vi "Config_Pulses_Tomography_v1.vi"(7 "init file iterator":u8, 8 "error in":errorcluster, 10 "Config files paths":T1={"ZI config file (.ini)"="Tomography_v1_config_dir\\Zurich_params.ini", "Keithley config file (.ini)"="Tomography_v1_config_dir\\Keithley_params.ini", "Arduino config file (.ini)"="Tomography_v1_config_dir\\pulse_sequence_dir\\"}, 11 "Resources in":T2 {"ZI ModHandle"."ModHandle" format="0x%08x"; "ZI ModHandle"."Conn" format="0x%08x"; "ZI Handle"."Handle" format="0x%08x"; "ZI Handle"."Conn" format="0x%08x"}) -> (0 "error out":errorcluster, 1 "Pulse sequence":T5[](array[typedef]) {"channel" min=2 max=13 step=1}, 2 "Init States":T8, 3 "Resources out":T2 {"ZI ModHandle"."ModHandle" format="0x%08x"; "ZI ModHandle"."Conn" format="0x%08x"; "ZI Handle"."Handle" format="0x%08x"; "ZI Handle"."Conn" format="0x%08x"}, 5 "Config files paths (single)":T1={"ZI config file (.ini)"="Config_Ver_1\\Zurich_params.ini", "Keithley config file (.ini)"="Config_Ver_1\\Keithley_params.ini", "Arduino config file (.ini)"="Config_Ver_1\\pulse_sequence.ini"})   [LabVIEW 2021]
uses:
  Ver_1/Config_File_Paths.ctl
  Ver_1/Resources.ctl
  <instrlib>/Zurich Instruments LabOne/Public/ziTypeHandle.ctl
  <instrlib>/Zurich Instruments LabOne/Public/Modules/ziTypeModHandle.ctl
  Drivers/Arduino_Pulse_Generator/Configurate/Register_1.ctl
  Drivers/Arduino_Pulse_Generator/Configurate/Register_2.ctl
  Drivers/Arduino_Pulse_Generator/Configurate/Channel_Pulse_Stream.ctl
  <instrlib>/Zurich Instruments LabOne/Zurich Instruments LabOne.lvlib
panel:
  out "String":string
  out "x-y":u32
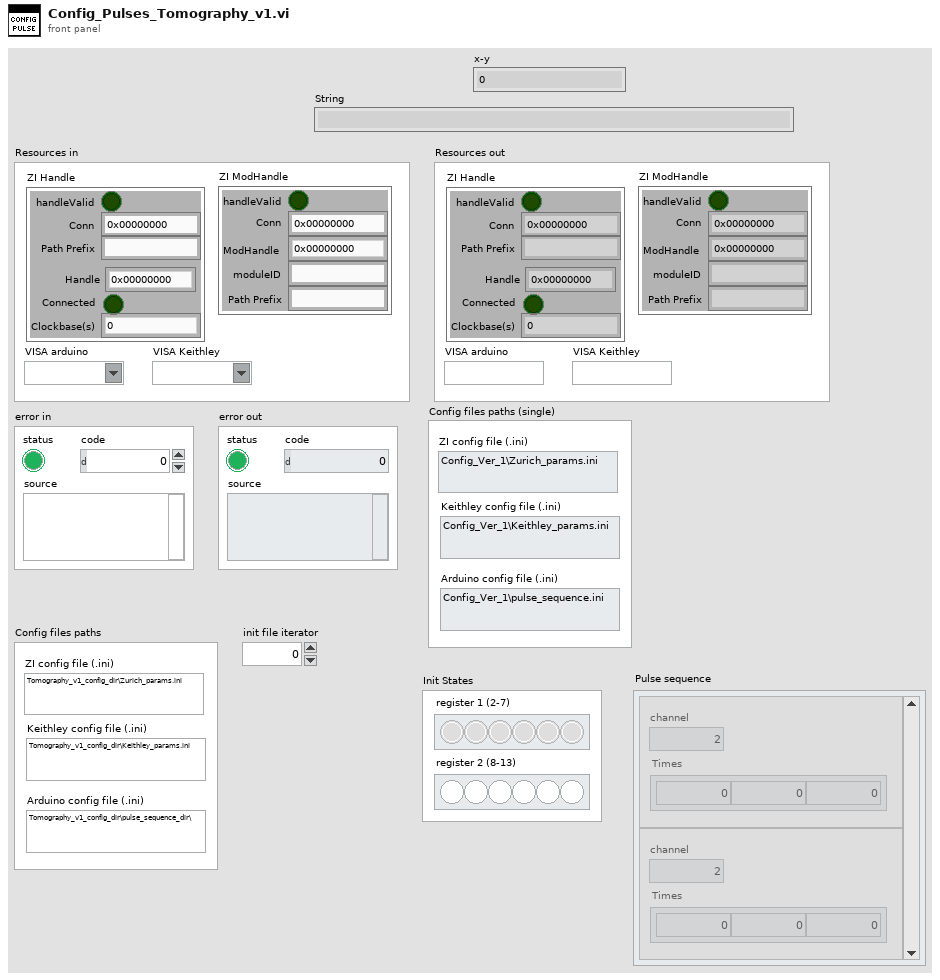
[diagram p1: front panel]
types:
  T1 = typedef "Config_File_Paths.ctl" = cluster{"ZI config file (.ini)":string, "Keithley config file (.ini)":string, "Arduino config file (.ini)":string}
  T2 = typedef "Resources.ctl" = cluster{"ZI Handle":T3, "ZI ModHandle":T4, "VISA arduino":refnum<visa-resource-name>, "VISA Keithley":refnum<visa-resource-name>}
  T3 = typedef "Zurich Instruments LabOne.lvlib/ziTypeHandle.ctl" = cluster{"handleValid":bool, "Conn":u64, "Path Prefix":string, "Handle":u64, "Connected":bool, "Clockbase(s)":dbl}
  T4 = typedef "Zurich Instruments LabOne.lvlib/ziTypeModHandle.ctl" = cluster{"handleValid":bool, "Conn":u64, "ModHandle":u64, "moduleID":string, "Path Prefix":string}
  T5 = typedef "Channel_Pulse_Stream.ctl" = cluster{"Times":dbl[], "channel":u8}
  T6 = typedef "Register_1.ctl" = bool[]
  T7 = typedef "Register_2.ctl" = bool[]
  T8 = cluster{"register 1 (2-7)":T6, "register 2 (8-13)":T7}
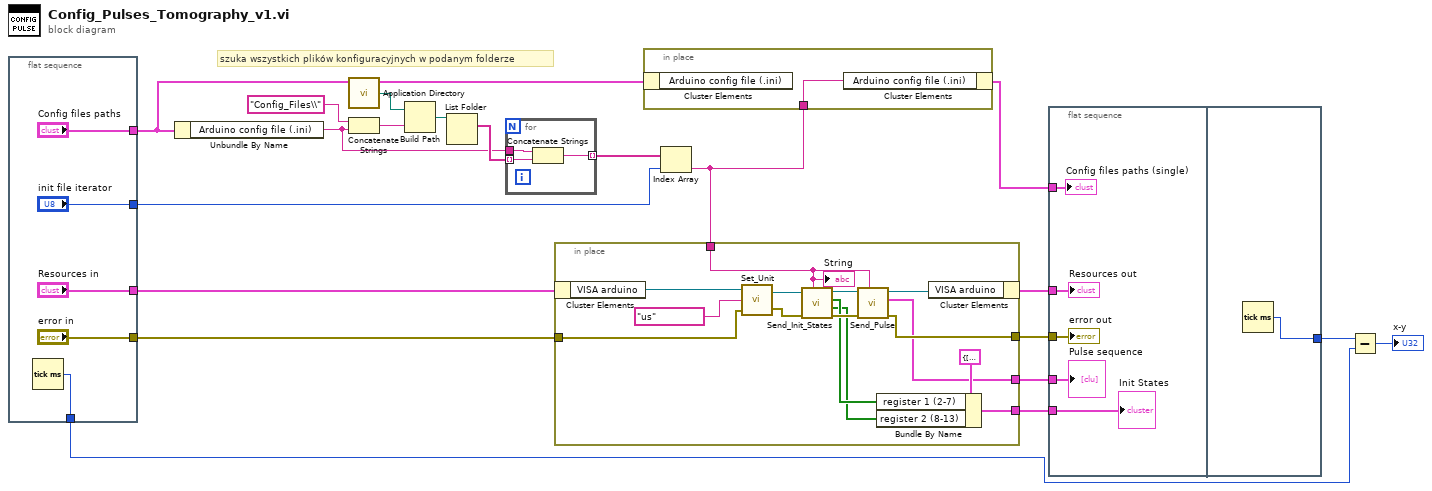
[diagram p0: block diagram]
diagram:
  # "szuka wszystkich plików konfiguracyjnych w podanym folderze"
  n1 = flat-sequence {
    tunnel: ["Config files paths"] -> w3
    tunnel: ["Resources in"] -> w14
    tunnel: ["init file iterator"] -> w12
    tunnel: ["error in"] -> w11
    tunnel: [w21] -> w5
    frame #0 {
      n2 = Tick Count (ms)() -> (millisecond timer value=w21:u32)
    }
  }
  n3 = Unbundle By Name(w3) -> ("Arduino config file (.ini)"=w16:string)
  n4 = call <vilib>:"Application Directory.vi"() -> ("Application Directory"=w20:path)
  n5 = Concatenate Strings("Config_Files\\" ("string"), w16) -> (w15:string)
  n6 = Build Path(base path=w20, name or relative path=w15) -> (appended path=w19:path)
  n7 = List Folder(path=w19) -> (filenames=w17:string[])  [unwired: 3 in, 3 out]
  n8 = for {
    tunnel: w17 -> [w28] mode=indexing
    tunnel: w16 -> [w27]
    tunnel: [w26] -> w13 mode=indexing
    n9 = Concatenate Strings(w27, w28) -> (w26:string)
  }
  n10 = Index Array(array=w13, index=w12) -> (element=w2:string)
  n11 = in-place {
    in-place-border: w2 -> [w34]
    in-place-border: w11 -> [w41]
    in-place-border: [w36] -> w7
    in-place-border: [w32] -> w10
    in-place-border: [w31] -> w9
    n12 = in-place-cluster #1(w14) -> ("VISA arduino"=w43:refnum<visa-resource-name>)
    n13 = call "Set_Unit.vi"("error in"=w41, "Unit"="us", "VISA arduino in"=w43) -> ("error out"=w35:errorcluster, "VISA arduino out"=w38:refnum<visa-resource-name>)
    n14 = call "Send_Init_States.vi"("Filename (.ini)"=w34, "error in"=w35, "VISA arduino in"=w38) -> ("error out"=w40:errorcluster, "register 2 (8-13)"=w29:T7, "register 1 (2-7)"=w30:T6, "VISA arduino out"=w39:refnum<visa-resource-name>)  [unwired: 5 in]
    n15 = call "Send_Pulse.vi"("Filename (.ini)"=w34, "error in"=w40, "VISA arduino in"=w39) -> ("error out"=w36:errorcluster, "Pulse sequence"=w32:T5[], "VISA arduino out"=w37:refnum<visa-resource-name>)  [unwired: 6 in]
    n16 = Bundle By Name(cluster=T8 {"register 1 (2-7)"=[], "register 2 (8-13)"=[FALSE, FALSE, FALSE, FALSE, FALSE, FALSE]} ("Init States"), "register 1 (2-7)"=w30, "register 2 (8-13)"=w29) -> (w31:T8)
    n17 = in-place-cluster #1("VISA arduino"=w37) -> (w8:T2)
    "String" <- w34
  }
  n18 = in-place {
    in-place-border: w2 -> [w44]
    n19 = in-place-cluster #2(w3) -> ()  [unwired: 1 out]
    n20 = in-place-cluster #2("Arduino config file (.ini)"=w44) -> (w1:T1)
  }
  n21 = flat-sequence {
    tunnel: w10 -> [w49]
    tunnel: w9 -> [w48]
    tunnel: w8 -> [w47]
    tunnel: w7 -> [w46]
    tunnel: w1 -> [w45]
    tunnel: [w50] -> w6
    frame #0 {
      "Pulse sequence" <- w49
      "Init States" <- w48
      "Resources out" <- w47
      "error out" <- w46
      "Config files paths (single)" <- w45
    }
    frame #1 {
      n22 = Tick Count (ms)() -> (millisecond timer value=w50:u32)
    }
  }
  n23 = Subtract(x=w6, y=w5) -> (x-y=→"x-y":u32)
